vi "T1 relaxometry Sequence Generator.vi"(5 "Optical Pulse":T1(array[cluster]), 7 "No. Instructions":i32, 8 "type":u16(ring) items=["Linear", "Logarithmic"], 9 "Rest time No. Steps":i32, 10 "Rest time Max":dbl=5e-07, 11 "Rest time Min":dbl=5e-08) -> (2 "Pulse Width":dbl[](array[numeric]), 3 "Pulse Sequence Out":T1(array[cluster]))   [LabVIEW 2012]
uses:
  <vilib>/Analysis/1siggen.llb/Ramp Pattern by Samples.vi
  <vilib>/Analysis/NI_AALBase.lvlib
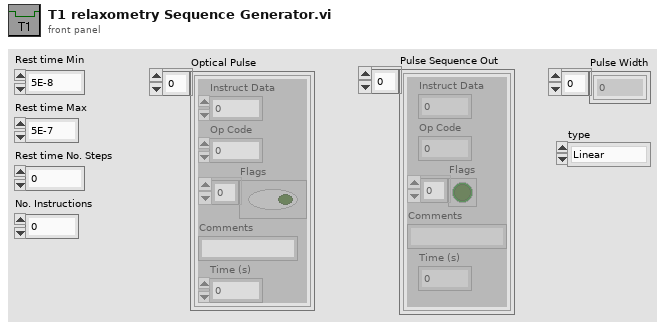
[diagram p1: front panel]
types:
  T1 = cluster{"Instruct Data":i32, "Op Code":i32, "Flags":bool[], "Comments":string, "Time (s)":dbl}[]
  T2 = cluster{"Instruct Data":i32, "Op Code":i32, "Flags":bool[], "Comments":string, "Time (s)":dbl}
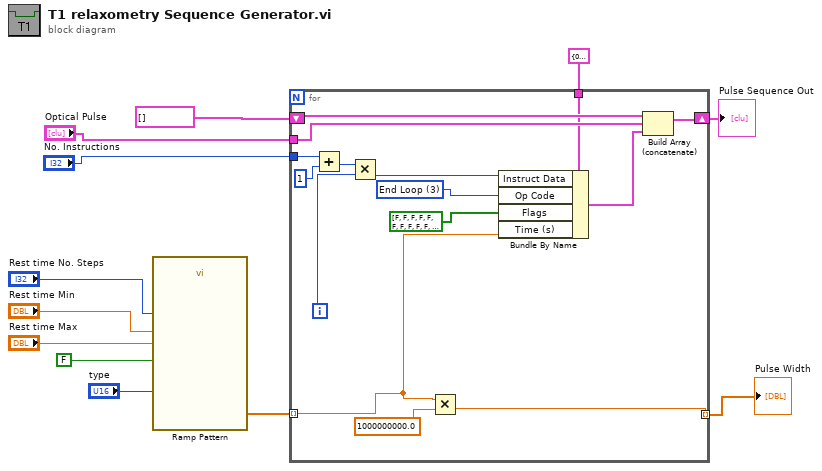
[diagram p0: block diagram]
diagram:
  n1 = call-poly <vilib>:"Ramp Pattern.vi"("type"="type", "exclude end?"=FALSE, "start"="Rest time Min", "end"="Rest time Max", "samples"="Rest time No. Steps") -> ("Ramp Pattern"=w3:dbl[])  [unwired: 5 in, 1 out]
  n2 = for {
    shift-right: [w26] -> w8
    shift-left: T1 [] -> [w27]
    tunnel: "Optical Pulse" -> [w24]
    tunnel: T2 {"Instruct Data"=0, "Op Code"=0, "Flags"=[FALSE, FALSE, FALSE, FALSE, FALSE, FALSE, FALSE, FALSE, FALSE, FALSE, FALSE, FALSE, FALSE, FALSE, FALSE, FALSE, FALSE, FALSE, FALSE, FALSE, FALSE, TRUE, TRUE, TRUE], "Comments"="", "Time (s)"=0.01} ("PB Inst 2") -> [w21]
    tunnel: [w17] -> w9 mode=indexing
    tunnel: "No. Instructions" -> [w16]
    tunnel: w3 -> [w13] mode=indexing
    i -> [w18]
    w23 = 3 items=["Continue", "Stop", "Loop", "End Loop", "JSR", "RTS", "Branch", "Long Delay", "Wait"] ("Op Code")
    n3 = Add(x=w16, y=1) -> (x+y=w19:i32)
    n4 = Multiply(x=w19, y=w18) -> (x*y=w15:i32)
    n5 = Multiply(x=w13, y=1000000000.0) -> (x*y=w17:dbl)
    n6 = Bundle By Name(cluster=w21, "Instruct Data"=w15, "Op Code"=w23, "Flags"=bool[] [FALSE, FALSE, FALSE, FALSE, FALSE, FALSE, FALSE, FALSE, FALSE, FALSE, FALSE, FALSE, FALSE, FALSE, FALSE, FALSE, FALSE, FALSE, FALSE, FALSE, FALSE, TRUE, TRUE, TRUE], "Time (s)"=w13) -> (w14:T2)
    n7 = Build Array (concatenate)(w27, w24, w14) -> (w26:T1)
  }
  "Pulse Width" <- w9
  "Pulse Sequence Out" <- w8
